vi "N-Channel 1-Sample (1D DBL).vi"() -> ()   [LabVIEW 2019]
uses:
  <vilib>/DAQmx/read.llb/DAQmx Read (Analog 1D DBL NChan 1Samp).vi
  <vilib>/DAQmx/create/channels.llb/DAQmx Create Channel (AI-Voltage-Basic).vi
  <vilib>/DAQmx/configure/timing.llb/DAQmx Timing (Sample Clock).vi
  <vilib>/DAQmx/miscellaneous.llb/DAQmx Fill In Error Info.vi
panel:
  in  "Stop":bool
  in  "Thermocouple Channel":tag
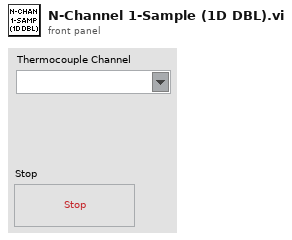
[diagram p1: front panel]
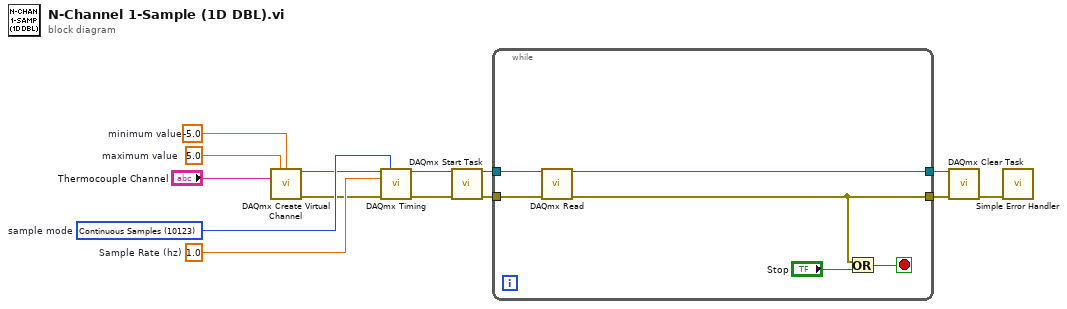
[diagram p0: block diagram]
diagram:
  w6 = 5.0  # maximum value
  w7 = -5.0  # minimum value
  w13 = 1.0  # Sample Rate (hz)
  w14 = 10123 items=["Finite Samples"=10178, "Continuous Samples"=10123, "Hardware Timed Single Point"=12522]  # sample mode
  n1 = call-poly <vilib>:"DAQmx Create Virtual Channel.vi"("maximum value"=w6, "minimum value"=w7, "physical channels"="Thermocouple Channel") -> ("task out"=w12:refnum<k21>, "error out"=w11:errorcluster)  [unwired: 11 in]
  n2 = call-poly <vilib>:"DAQmx Timing.vi"("task/channels in"=w12, "sample mode"=w14, "rate"=w13, "error in"=w11) -> ("task out"=w10:refnum<k21>, "error out"=w9:errorcluster)  [unwired: 10 in]
  n3 = call <vilib>:"DAQmx Start Task.vi"("task/channels in"=w10, "error in"=w9) -> ("task out"=w2:refnum<k21>, "error out"=w1:errorcluster)  [unwired: 12 in]
  n4 = while {
    tunnel: [w20] -> w5
    tunnel: [w19] -> w4
    tunnel: w2 -> [w16]
    tunnel: w1 -> [w15]
    stop <- w17 stop-if-true
    n5 = call-poly <vilib>:"DAQmx Read.vi"("task/channels in"=w16, "error in"=w15) -> ("task out"=w20:refnum<k21>, "error out"=w19:errorcluster)  [unwired: 11 in, 1 out]
    n6 = Or(x=w19, y="Stop") -> (x .or. y?=w17:bool)
  }
  n7 = call <vilib>:"DAQmx Clear Task.vi"("task in"=w5, "error in"=w4) -> ("error out"=w3:errorcluster)  [unwired: 13 in]
  n8 = call <vilib>:"Simple Error Handler.vi"("error in (no error)"=w3) -> ()  [unwired: 4 in, 5 out]
